vi "Oscop Phase Read Averaging.vi"(8 "error in (no error)":errorcluster, 10 "Numeric in":i32, 11 "VISA Refnum in":refnum<visa-resource-name>) -> (0 "error out":errorcluster, 2 "Numeric out":dbl, 3 "VISA Refnum out":refnum<visa-resource-name>)   [LabVIEW 2021]
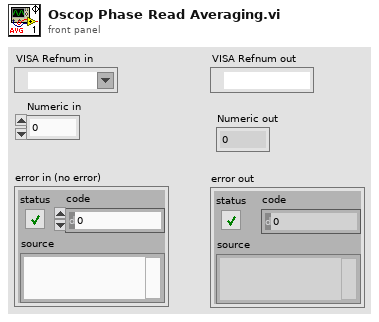
[diagram p1: front panel]
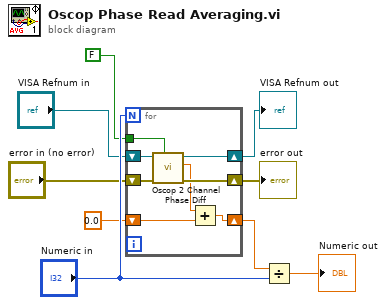
[diagram p0: block diagram]
diagram:
  n1 = for {
    N: "Numeric in" -> [_]
    tunnel: FALSE ("Perform Auto Setup") -> [w10]
    shift-right: [w13] -> w3
    shift-left: "error in (no error)" -> [w12]
    shift-right: [w14] -> w6
    shift-left: "VISA Refnum in" -> [w15]
    shift-right: [w17] -> w9
    shift-left: 0.0 -> [w16]
    n2 = call "Oscop 2 Channel Phase Diff.vi"("Perform Auto Setup"=w10, "error in (no error)"=w12, "VISA resource name"=w15) -> ("error out"=w13:errorcluster, "Value"=w11:dbl, "VISA resource name out"=w14:refnum<visa-resource-name>)  [unwired: 6 in]
    n3 = Add(x=w11, y=w16) -> (x+y=w17:dbl)
  }
  "VISA Refnum out" <- w6
  "error out" <- w3
  n4 = Divide(x=w9, y="Numeric in") -> (x/y=→"Numeric out":dbl)
